vi "Get Cell.vi"(8 "error in":errorcluster, 10 "Cell Address":string="A", 11 "Row in":refnum<k24>) -> (0 "error out":errorcluster, 2 "Cell":refnum<k24>, 3 "Row out":refnum<k24>)   [LabVIEW 2021, in "Open Xml.lvlib"]
doc: "Returns Cell with specified address if existing."
uses:
  Open Xml.lvlib
  D:/git/Open-Xml-LabVIEW/dll/DocumentFormat.OpenXml.dll
  dll/DocumentFormat.OpenXml.dll
  D:/git/Open-Xml-LabVIEW/dll/DocumentFormat.OpenXml.Framework.dll
  dll/DocumentFormat.OpenXml.Framework.dll
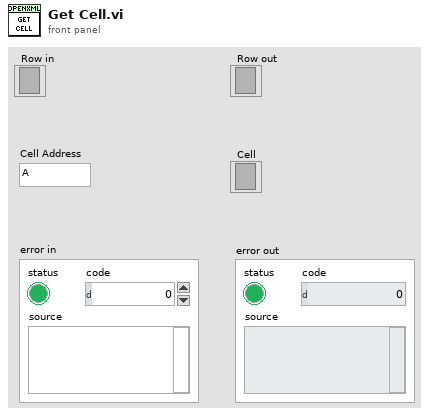
[diagram p1: front panel]
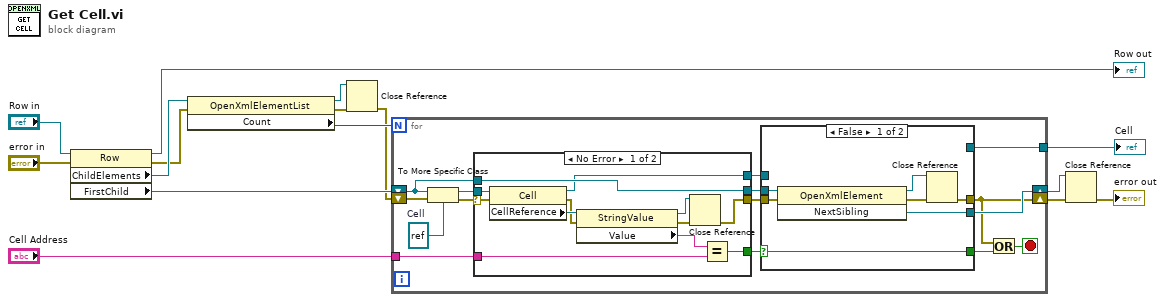
[diagram p0: block diagram]
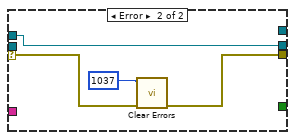
[diagram p2: hidden frame]
diagram:
  n1 = property class="Row"(reference="Row in", error in="error in") -> (reference out=→"Row out":refnum<k24>, error out=w7:errorcluster, "ChildElements"=w15:refnum<k24>, "FirstChild"=w13:refnum<k24>)
  n2 = property class="OpenXmlElementList"(reference=w15, error in=w7) -> (reference out=w10:refnum<k24>, error out=w9:errorcluster, "Count"=w14:i32)
  n3 = Close Reference(reference=w10, error in (no error)=w9) -> (error out=w8:errorcluster)
  n4 = for {
    N: w14 -> [_]
    shift-right: [w21] -> w11
    shift-left: w13 -> [w27]
    tunnel: "Cell Address" -> [w25]
    tunnel: [w17] -> w1
    shift-right: [w20] -> w12
    shift-left: w8 -> [w29]
    stop <- w24 stop-if-true
    w30 = refnum<k24> refnum  # Cell
    n5 = To More Specific Class(target class=w30, reference=w27, error in=w29) -> (specific class reference=w26:refnum<k24>, error out=w28:errorcluster)
    n6 = case shown="No Error" w28 {
      selector: w28 -> [w42 w46]
      tunnel: [w31 w44] -> w23
      tunnel: w27 -> [w36 w45]
      tunnel: [w36 w45] -> w22
      tunnel: [w37 _] -> w16
      tunnel: w26 -> [w41 _]
      tunnel: w25 -> [w38 _]
      tunnel: [w35 _] -> w18
      frame No Error {
        n7 = property class="Cell"(reference=w41, error in=w42) -> (reference out=w35:refnum<k24>, error out=w34:errorcluster, "CellReference"=w40:refnum<k24>)
        n8 = property class="StringValue"(reference=w40, error in=w34) -> (reference out=w32:refnum<k24>, error out=w33:errorcluster, "Value"=w39:string)
        n9 = Close Reference(reference=w32, error in (no error)=w33) -> (error out=w31:errorcluster)
        n10 = Equal?(x=w39, y=w38) -> (x = y?=w37:bool)
      }
      frame Error {
        n11 = call <vilib>:"Clear Errors.vi"("error in (no error)"=w46, "specific error code to clear (0: all)"=1037) -> ("error out"=w44:errorcluster)  [unwired: 4 in, 1 out]
      }
    }
    n12 = case shown="False" w16 {
      selector: w16 -> [w47 w56]
      tunnel: w23 -> [w53 w55]
      tunnel: w22 -> [w51 _]
      tunnel: [w50 _] -> w21
      tunnel: [w48 w55] -> w20
      tunnel: [w47 w56] -> w19
      tunnel: w18 -> [_ w54]
      tunnel: [_ w54] -> w17
      frame False {
        n13 = invoke class="OpenXmlElement" method="NextSibling"(reference=w51, error in=w53) -> (reference out=w49:refnum<k24>, error out=w52:errorcluster, "NextSibling"=w50:refnum<k24>)  [unwired: 1 in]
        n14 = Close Reference(reference=w49, error in (no error)=w52) -> (error out=w48:errorcluster)
      }
      frame True {
      }
    }
    n15 = Or(x=w20, y=w19) -> (x .or. y?=w24:bool)
  }
  "Cell" <- w1
  n16 = Close Reference(reference=w11, error in (no error)=w12) -> (error out=→"error out":errorcluster)
